vi "[FP] - Place on Point Size to Decoration.vi"(7 "Point":T1, 8 "Error":errorcluster, 9 "FPSet":T2={"Menu Bar"=FALSE, "Position"=enum."MID-CTR", "border(px)"=-2, "Monitor #"=0}, 11 "VI Ref":refnum<vi>) -> (0 "Error Out":errorcluster, 3 "VI Ref Out":refnum<vi>)   [LabVIEW 2015]
doc: "sets up a fp to center of monitor 1 around largest decoration. shows scroll bars if developing and hides them if not."
uses:
  TypeDefs_Utility/Cluster_FP_Position  and Size Data.ctl
  TypeDefs_Utility/ENUM RB_Pos_Quadrant Position.ctl
  TypeDefs_Utility/Cluster_Pos_Top Left position.ctl
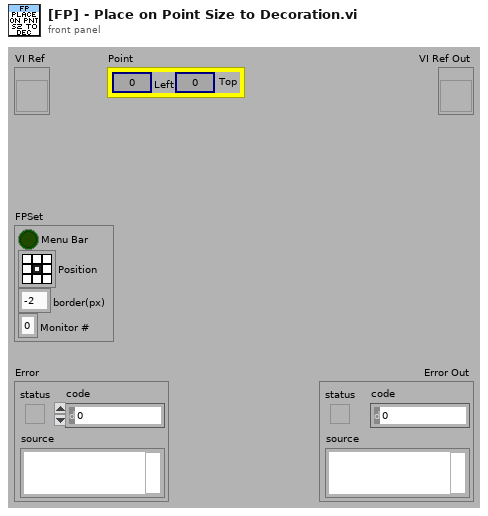
[diagram p1: front panel]
types:
  T1 = typedef "Cluster_Pos_Top Left position.ctl" = cluster{"Left":i16, "Top":i16}
  T2 = typedef "Cluster_FP_Position  and Size Data.ctl" = cluster{"Menu Bar":bool, "Position":T3, "border(px)":i32, "Monitor #":u16}
  T3 = typedef "ENUM RB_Pos_Quadrant Position.ctl" = enum32{"LFT-TOP", "MID-TOP", "RGT-TOP", "LFT-CTR", "MID-CTR", "RGT-CTR", "LFT-BOT", "MID-BOT", "RGT-BOT"}
  T4 = enum32{"invalid app kind", "Development System", "Run Time System", "Student Edition", "Embedded LabVIEW", "Evaluation", "Custom"}
  T5 = enum32{"Invalid", "Standard", "Closed", "Hidden", "Minimized", "Maximized"}
  T6 = enum16{"Always On", "Always Off", "Off While Running"}
  T7 = typedef "LVRectTypeDef.ctl" = cluster{"Left":i16, "Top":i16, "Right":i16, "Bottom":i16}
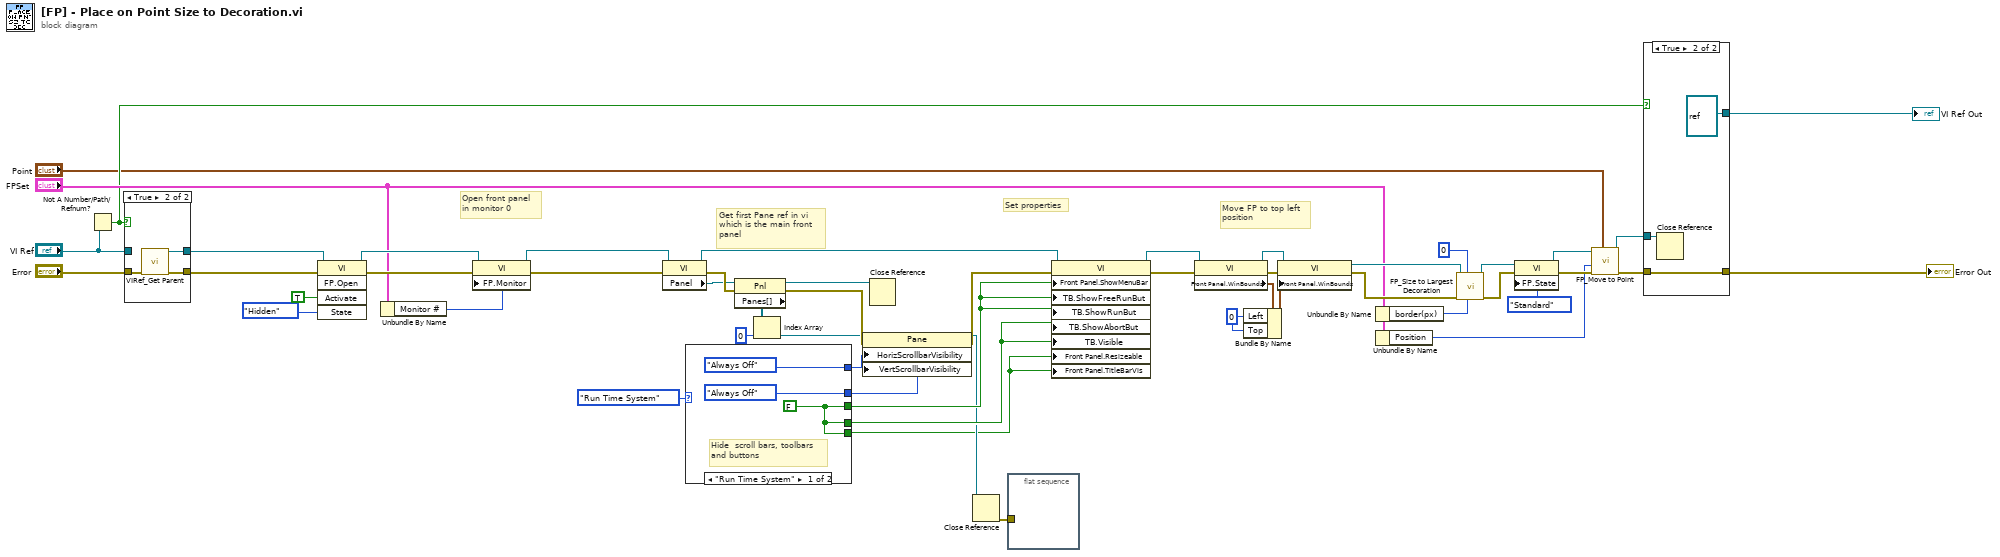
[diagram p0: block diagram]
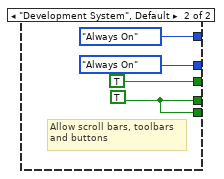
[diagram p4: hidden frame]
diagram:
  w33 = i16 0 ("left")
  # "Move FP to top left\nposition"
  # "Set properties"
  # "Get first Pane ref in vi\nwhich is the main front\npanel"
  # "Open front panel\nin monitor 0"
  n1 = Not A Number/Path/Refnum?(number/path/refnum="VI Ref") -> (NaN/Path/Refnum?=w4:bool)
  n2 = case shown="True" w4 {
    tunnel: [w54 w57] -> w11
    tunnel: "VI Ref" -> [w54 _]
    tunnel: [w53 w55] -> w9
    tunnel: "Error" -> [w53 w56]
    frame False {
    }
    frame True {
      n3 = call "VIRef_Get Parent.vi"("error in (no error)"=w56) -> ("VI Refnum"=w57:refnum<vi>, "error out"=w55:errorcluster)  [unwired: 16 in, 1 out]
    }
  }
  n4 = invoke class="VI" method="FP.Open"(reference=w11, error in=w9, "Activate"=TRUE ("Front Panel Window:Open"), "State"=T5."Hidden" ("Front Panel Window:State")) -> (reference out=w18:refnum<vi>, error out=w17:errorcluster)  [unwired: 1 in, 3 out]
  n5 = Unbundle By Name("FPSet") -> ("Monitor #"=w13:u16)
  n6 = property class="VI"(reference=w18, error in=w17, "FP.Monitor"=w13) -> (reference out=w28:refnum<vi>, error out=w29:errorcluster)
  n7 = property class="VI"(reference=w28, error in=w29) -> (reference out=w40:refnum<vi>, error out=w49:errorcluster, "Panel"=w45:refnum<vi>)
  n8 = case shown="\"Run Time System\"" T4."Run Time System" ("App.Kind") {
    tunnel: [T6."Always Off" ("Horizontal Scrollbar Visibility") T6."Always On" ("Horizontal Scrollbar Visibility")] -> w51
    tunnel: [w58 TRUE ("Front Panel Window:Show Menu Bar")] -> w24
    tunnel: [w58 w61] -> w42
    tunnel: [T6."Always Off" ("Horizontal Scrollbar Visibility") T6."Always On" ("Horizontal Scrollbar Visibility")] -> w41
    tunnel: [w58 w61] -> w19
    frame "Run Time System" {
      w58 = FALSE ("Front Panel Window:Show Menu Bar")
      # "Hide  scroll bars, toolbars\nand buttons"
    }
    frame "Development System", Default {
      w61 = TRUE ("Front Panel Window:Show Menu Bar")
      # "Allow scroll bars, toolbars\nand buttons"
    }
  }
  n9 = property class="Pnl"(reference=w45, error in=w49) -> (reference out=w43:refnum<vi>, error out=w48:errorcluster, "Panes[]"=w46:refnum<vi>[])
  n10 = Index Array(array=w46, index=0) -> (element=w47:refnum<vi>)
  n11 = property class="Pane"(reference=w47, error in=w48, "HorizScrollbarVisibility"=w41, "VertScrollbarVisibility"=w51) -> (reference out=w22:refnum<vi>, error out=w52:errorcluster)
  n12 = Close Reference(reference=w43) -> ()  [unwired: 1 in, 1 out]
  n13 = Close Reference(reference=w22) -> (error out=w27:errorcluster)  [unwired: 1 in]
  n14 = flat-sequence {
    tunnel: w27 -> [_]
    frame #0 {
    }
  }
  n15 = property class="VI"(reference=w40, error in=w52, "Front Panel.ShowMenuBar"=w24, "TB.ShowFreeRunBut"=w24, "TB.ShowRunBut"=w24, "TB.ShowAbortBut"=w42, "TB.Visible"=w42, "Front Panel.Resizeable"=w19, "Front Panel.TitleBarVis"=w19) -> (reference out=w39:refnum<vi>, error out=w37:errorcluster)
  n16 = property class="VI"(reference=w39, error in=w37) -> (reference out=w38:refnum<vi>, error out=w36:errorcluster, "Front Panel.WinBounds"=w35:T7)
  n17 = Bundle By Name(cluster=w35, "Left"=w33, "Top"=w33) -> (w34:T7)
  n18 = property class="VI"(reference=w38, error in=w36, "Front Panel.WinBounds"=w34) -> (reference out=w30:refnum<vi>, error out=w31:errorcluster)
  n19 = Unbundle By Name("FPSet") -> ("border(px)"=w25:i32)
  n20 = Unbundle By Name("FPSet") -> ("Position"=w2:T3)
  n21 = call "FP_Size to Largest Decoration.vi"("Border Spacing (2 Px)"=w25, "Decoration index"=0, "Error"=w31, "VI Ref"=w30) -> ("Error Out"=w23:errorcluster, "VI Ref Out"=w32:refnum<vi>)  [unwired: 2 in, 4 out]
  n22 = property class="VI"(reference=w32, error in=w23, "FP.State"=T5."Standard" ("Front Panel Window:State")) -> (reference out=w26:refnum<vi>, error out=w21:errorcluster)
  n23 = call "FP_Move to Point.vi"("Target Point"="Point", "Error"=w21, "FP Position"=w2, "VI"=w26) -> ("Error Out"=w8:errorcluster, "VI Out"=w6:refnum<vi>)  [unwired: 6 in]
  n24 = case shown="True" w4 {
    tunnel: w6 -> [w66 w69]
    tunnel: w8 -> [w65 w67]
    tunnel: [w65 w67] -> w7
    tunnel: [w66 refnum<vi> refnum ("Vi Ref (this Vi) Out")] -> w5
    frame False {
    }
    frame True {
      n25 = Close Reference(reference=w69) -> ()  [unwired: 1 in, 1 out]
    }
  }
  "Error Out" <- w7
  "VI Ref Out" <- w5
